vi "Write B.vi"(8 "error in (no error)":errorcluster, 10 "fieldB":string, 11 "My Custom Type in":refnum<class "My Custom Type.lvclass">) -> (0 "error out":errorcluster, 3 "My Custom Type out":refnum<class "My Custom Type.lvclass">)   [LabVIEW 2020, in "My Custom Type.lvclass"]
uses:
  My Custom Type.lvclass
  My Custom Type.lvclass/My Custom Type.ctl
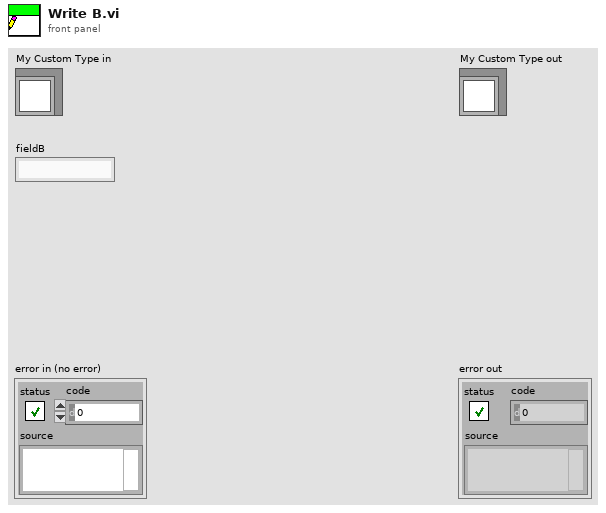
[diagram p1: front panel]
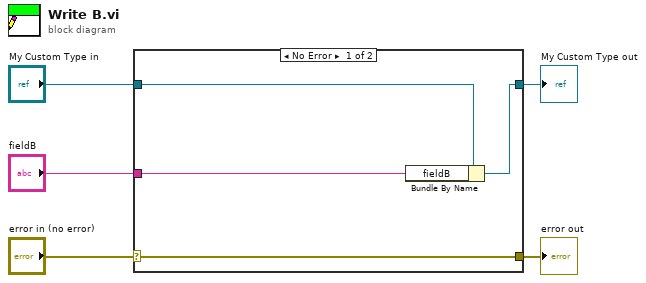
[diagram p0: block diagram]
diagram:
  n1 = case shown="No Error" "error in (no error)" {
    selector: "error in (no error)" -> [w9 w10]
    tunnel: [w9 w10] -> w4
    tunnel: [w7 w11] -> w2
    tunnel: "My Custom Type in" -> [w8 w11]
    tunnel: "fieldB" -> [w6 _]
    frame No Error {
      n2 = Bundle By Name(cluster=w8, "fieldB"=w6) -> (w7:refnum<class "My Custom Type.lvclass">)
    }
    frame Error {
    }
  }
  "error out" <- w4
  "My Custom Type out" <- w2
